vi "SwerveMath.vi"(0 "X-Axis":dbl, 2 "Y-Axis":dbl, 4 "Turn":dbl) -> (20 "FrontLeftTarget":dbl, 21 "FrontRightTarget":dbl, 22 "RearLeftTarget":dbl, 23 "RearRightTarget":dbl, 24 "FrontLeftDrive":dbl, 25 "FrontRightDrive":dbl, 26 "RearLeftDrive":dbl, 27 "RearRightDrive":dbl)   [LabVIEW 2017]
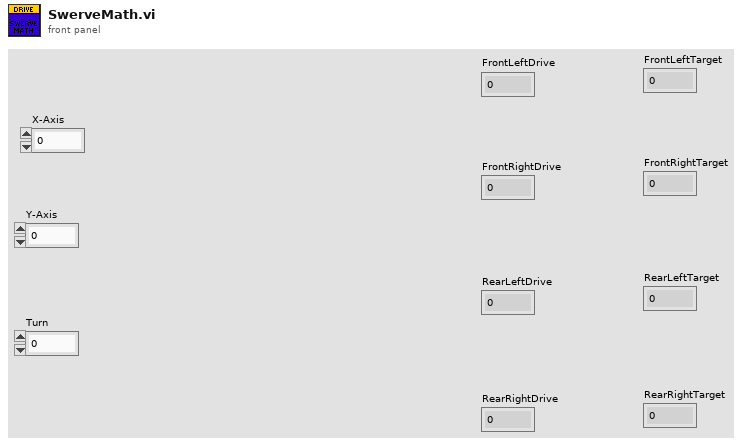
[diagram p1: front panel]
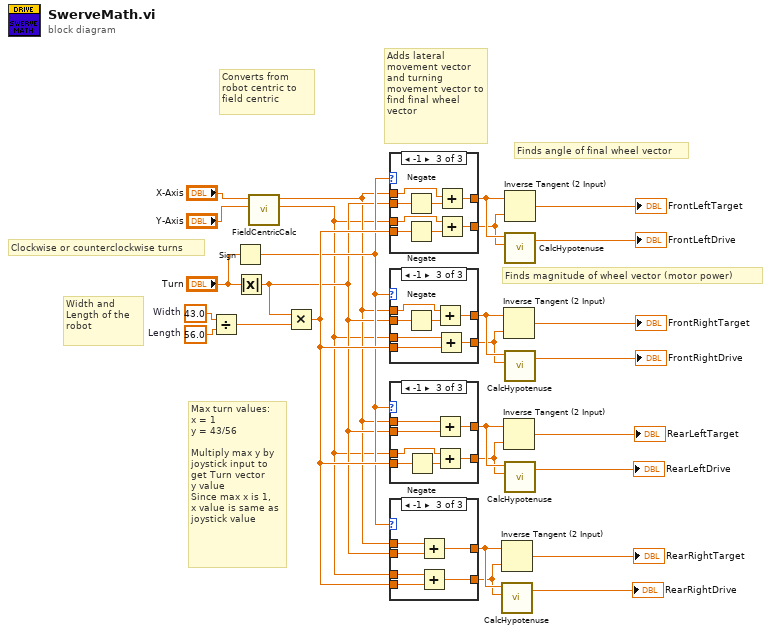
[diagram p0: block diagram]
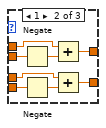
[diagram p3: hidden frame]
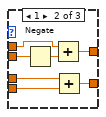
[diagram p5: hidden frame]
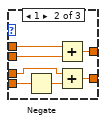
[diagram p7: hidden frame]
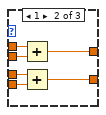
[diagram p9: hidden frame]
diagram:
  w26 = 56.0  # Length
  w27 = 43.0  # Width
  # "Finds magnitude of wheel vector (motor power)"
  # "Finds angle of final wheel vector"
  # "Adds lateral movement vector and turning movement vector to find final wheel vector"
  # "Width and Length of the robot"
  # "Converts from robot centric to field centric"
  # "Clockwise or counterclockwise turns"
  # "Max turn values:\nx = 1\ny = 43/56\n\nMultiply max y by\njoystick input to\nget Turn vector\ny value\nSince max x is 1,\nx value is same as\njoystick value"
  n1 = Divide(x=w27, y=w26) -> (x/y=w24:dbl)
  n2 = Sign(1:"Turn") -> (0:w13:dbl)
  n3 = Absolute Value(x="Turn") -> (abs(x)=w9:dbl)
  n4 = call "FieldCentricCalc.vi"("y_in"="Y-Axis", "x_in"="X-Axis") -> ("y_out"=w1:dbl, "x_out"=w2:dbl)  [unwired: 8 in]
  n5 = Multiply(x=w9, y=w24) -> (x*y=w25:dbl)
  n6 = case shown="-1" w13 {
    tunnel: [w29 w35 w43] -> w17
    tunnel: [w28 w34 w42] -> w16
    tunnel: w2 -> [w29 w33 w36]
    tunnel: w1 -> [w28 w32 w41]
    tunnel: w25 -> [_ w31 w38]
    tunnel: w9 -> [_ w30 w39]
    frame 0, Default {
    }
    frame 1 {
      n7 = Add(x=w33, y=w30) -> (x+y=w35:dbl)
      n8 = Add(x=w32, y=w31) -> (x+y=w34:dbl)
    }
    frame -1 {
      n9 = Negate(x=w39) -> (-x=w40:dbl)
      n10 = Negate(x=w38) -> (-x=w37:dbl)
      n11 = Add(x=w36, y=w40) -> (x+y=w43:dbl)
      n12 = Add(x=w41, y=w37) -> (x+y=w42:dbl)
    }
  }
  n13 = case shown="-1" w13 {
    tunnel: [w45 w52 w59] -> w15
    tunnel: [w44 w51 w58] -> w14
    tunnel: w2 -> [w45 w50 w56]
    tunnel: w1 -> [w44 w49 w55]
    tunnel: w25 -> [_ w47 w54]
    tunnel: w9 -> [_ w48 w53]
    frame 0, Default {
    }
    frame 1 {
      n14 = Negate(x=w47) -> (-x=w46:dbl)
      n15 = Add(x=w50, y=w48) -> (x+y=w52:dbl)
      n16 = Add(x=w49, y=w46) -> (x+y=w51:dbl)
    }
    frame -1 {
      n17 = Negate(x=w53) -> (-x=w57:dbl)
      n18 = Add(x=w56, y=w57) -> (x+y=w59:dbl)
      n19 = Add(x=w55, y=w54) -> (x+y=w58:dbl)
    }
  }
  n20 = case shown="-1" w13 {
    tunnel: [w61 w68 w75] -> w20
    tunnel: [w60 w67 w74] -> w19
    tunnel: w2 -> [w61 w65 w73]
    tunnel: w1 -> [w60 w64 w72]
    tunnel: w25 -> [_ w63 w70]
    tunnel: w9 -> [_ w62 w71]
    frame 0, Default {
    }
    frame 1 {
      n21 = Negate(x=w62) -> (-x=w66:dbl)
      n22 = Add(x=w65, y=w66) -> (x+y=w68:dbl)
      n23 = Add(x=w64, y=w63) -> (x+y=w67:dbl)
    }
    frame -1 {
      n24 = Negate(x=w70) -> (-x=w69:dbl)
      n25 = Add(x=w73, y=w71) -> (x+y=w75:dbl)
      n26 = Add(x=w72, y=w69) -> (x+y=w74:dbl)
    }
  }
  n27 = case shown="-1" w13 {
    tunnel: [w77 w85 w91] -> w23
    tunnel: [w76 w84 w90] -> w22
    tunnel: w2 -> [w77 w80 w88]
    tunnel: w1 -> [w76 w81 w89]
    tunnel: w25 -> [_ w79 w86]
    tunnel: w9 -> [_ w78 w87]
    frame 0, Default {
    }
    frame 1 {
      n28 = Negate(x=w78) -> (-x=w83:dbl)
      n29 = Negate(x=w79) -> (-x=w82:dbl)
      n30 = Add(x=w80, y=w83) -> (x+y=w85:dbl)
      n31 = Add(x=w81, y=w82) -> (x+y=w84:dbl)
    }
    frame -1 {
      n32 = Add(x=w88, y=w87) -> (x+y=w91:dbl)
      n33 = Add(x=w89, y=w86) -> (x+y=w90:dbl)
    }
  }
  n34 = Inverse Tangent (2 Input)(1:w22, 2:w23) -> (0:→"RearRightTarget":dbl)
  n35 = call "CalcHypotenuse.vi"("b"=w22, "a"=w23) -> ("hypotenuse"=→"RearRightDrive":dbl)  [unwired: 3 in]
  n36 = Inverse Tangent (2 Input)(1:w14, 2:w15) -> (0:→"FrontRightTarget":dbl)
  n37 = Inverse Tangent (2 Input)(1:w19, 2:w20) -> (0:→"RearLeftTarget":dbl)
  n38 = Inverse Tangent (2 Input)(1:w16, 2:w17) -> (0:→"FrontLeftTarget":dbl)
  n39 = call "CalcHypotenuse.vi"("b"=w16, "a"=w17) -> ("hypotenuse"=→"FrontLeftDrive":dbl)  [unwired: 3 in]
  n40 = call "CalcHypotenuse.vi"("b"=w14, "a"=w15) -> ("hypotenuse"=→"FrontRightDrive":dbl)  [unwired: 3 in]
  n41 = call "CalcHypotenuse.vi"("b"=w19, "a"=w20) -> ("hypotenuse"=→"RearLeftDrive":dbl)  [unwired: 3 in]
